vi "Lab1_A3_mainVI.vi"() -> ()   [LabVIEW 2020]
panel:
  in  "Signal Type":u16(ring) items=["square", "triangle", "sinusoidal"]
  in  "Amplitude":dbl
  in  "f(frequency of signal)":dbl
  in  "fs(sampling frequency)":dbl
  out "Waveform Chart":dbl(graph)
  in  "stop":bool
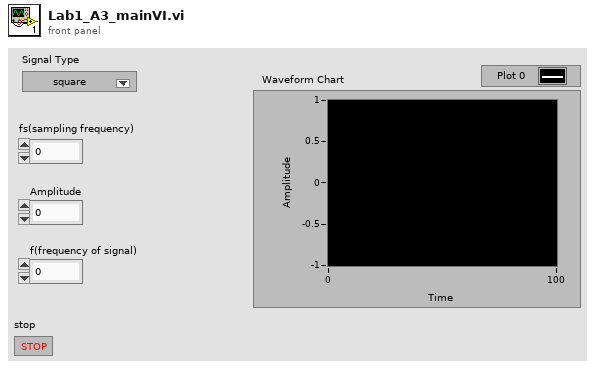
[diagram p1: front panel]
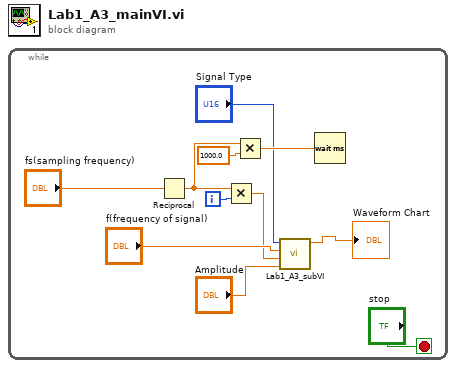
[diagram p0: block diagram]
diagram:
  n1 = while {
    i -> [w7]
    stop <- "stop" stop-if-true
    n2 = Reciprocal(x="fs(sampling frequency)") -> (1/x=w6:dbl)
    n3 = Multiply(x=w6, y=w7) -> (x*y=w3:dbl)
    n4 = Multiply(x=w6, y=1000.0) -> (x*y=w8:dbl)
    n5 = call "Lab1_A3_subVI.vi"("Amplitude"="Amplitude", "Time"=w3, "Frequency"="f(frequency of signal)", "Signal Type"="Signal Type") -> ("Signal"=→"Waveform Chart":dbl)  [unwired: 6 in]
    n6 = Wait (ms)(milliseconds to wait=w8) -> ()  [unwired: 1 out]
  }
